vi "SRS cleanup.vi"(8 "error in (no error)":errorcluster, 11 "RUS settings":T1={"NI-DAQ lockin settings"={"Samples per sine wave"=0, "Sine waves per freq step"=0, "Output Representation"=enum."Real/Imaginary", "Low-pass filter"=enum."Butterworth", "Ranges and couplings "=[]}, "Fast swep settings"={"Update rate (Hz)"=250.0, "Start F, Hz"=200000.0, "Stop F"=1700000.0, "Number of points"=30000, "Amplitude"=2.1, "Init&amplitude"=TRUE, "IF"=1000.0, "Time constant"=0.1}, "Pre-sweep delay, s"=0.0, "Lockin mode"=enum."NI-DAQ", "SR Lockin"="GPIB0::10::INSTR", "DAQmx Device"="Dev3", "Clock Multiplier"=64, "Fast Sweep Data Out"={"DO clock task"="", "DO task"="", "Update clock task"="", "DAQ lockin task"="", "Pre-sweep counter task"=""}, "Lockin Range, V"=0.0, "F Array"=[], "Freq. update clock terminal"="", "DO Clock Rate (Hz)"=5000000.0, "ADC clock terminal"="/PFI4", "Pre-sweep counter terminal"="/PFI4", "Samples per read"=10, "DO clock terminal"="", "Pre-sweep points"=0, "F points per write"=0, "Total sweep time, s"=1000.0, "Initial SYNTH phase"=0.0, "Record IF"=FALSE, "Save data settings"={"Save data"=TRUE, "Data Root Path"=path "", "File Prefix"="", "File Format"=enum."ASCII", "Save column names"=TRUE, "File Comments"="<Description of the current file>", "User/Prj"="<User Name/Project Description>"}, "Data file path"=path "", "New data user event"=refnum, "Stop user event"=refnum, "Number of channels"=1, "Auto-phase"=FALSE} {"Lockin Range, V" format="%#_6e"; "Fast swep settings"."IF" format="%#_6p"; "Fast swep settings"."Amplitude" min=0.0 max=2.5; "Fast swep settings"."Number of points" format="%.0p"; "Fast swep settings"."Stop F" format="%#_6p"; "Fast swep settings"."Start F, Hz" format="%#_6p"; "Fast swep settings"."Update rate (Hz)" format="%0.2f"; "NI-DAQ lockin settings"."Ranges and couplings"."Coupling" items=["default"=-1, "RSE"=10083, "NRSE"=10078, "Differential"=10106, "Pseudodifferential"=12529]}) -> (0 "error out":errorcluster, 3 "VISA resource name out":refnum<visa-resource-name>, 4 "STD status byte":u8 format="%08b", 5 "Error status byte\n(bit 5 - FAST aborted)":u8 format="%08b")   [LabVIEW 2015]
uses:
  resonant_ultrasound/Libraries/RUS/Controls/RUS settings.ctl
  resonant_ultrasound/Libraries/RUS/Controls/RUS NI-DAQ Lockin Settings.ctl
  resonant_ultrasound/Libraries/RUS/Controls/Sweep settings.ctl
  File/Controls/Save data settings.ctl
  File/Controls/File formats.ctl
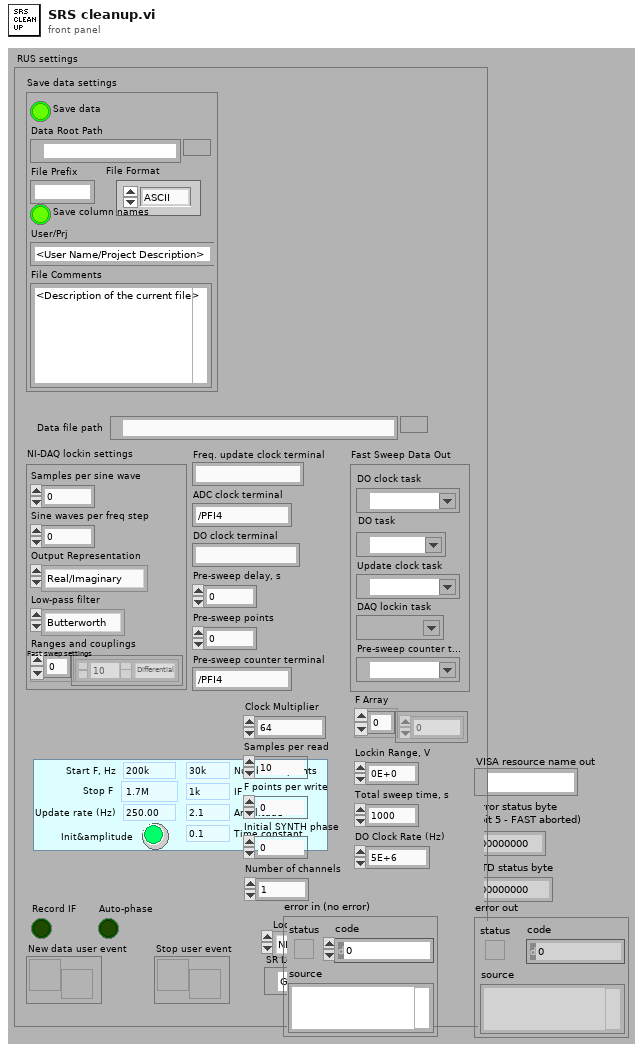
[diagram p1: front panel]
types:
  T1 = typedef "RUS settings.ctl" = cluster{"NI-DAQ lockin settings":T2, "Fast swep settings":T3, "Pre-sweep delay, s":dbl, "Lockin mode":enum16{"SRS", "NI-DAQ"}, "SR Lockin":refnum<visa-resource-name>, "DAQmx Device":tag, "Clock Multiplier":i32, "Fast Sweep Data Out":cluster{"DO clock task":refnum<k21>, "DO task":refnum<k21>, "Update clock task":refnum<k21>, "DAQ lockin task":refnum<k21>, "Pre-sweep counter task":refnum<k21>}, "Lockin Range, V":sgl, "F Array":dbl[], "Freq. update clock terminal":string, "DO Clock Rate (Hz)":dbl, "ADC clock terminal":string, "Pre-sweep counter terminal":string, "Samples per read":i32, "DO clock terminal":string, "Pre-sweep points":i32, "F points per write":i32, "Total sweep time, s":dbl, "Initial SYNTH phase":dbl, "Record IF":bool, "Save data settings":T4, "Data file path":path, "New data user event":refnum<user-event>, "Stop user event":refnum<user-event>, "Number of channels":i32, "Auto-phase":bool}
  T2 = typedef "RUS NI-DAQ Lockin Settings.ctl" = cluster{"Samples per sine wave":i32, "Sine waves per freq step":i32, "Output Representation":enum16{"Real/Imaginary", "Polar"}, "Low-pass filter":enum16{"No filtering", "Butterworth", "Bessel"}, "Ranges and couplings ":cluster{"Range":dbl, "Coupling":i32}[]}
  T3 = typedef "Sweep settings.ctl" = cluster{"Update rate (Hz)":dbl, "Start F, Hz":dbl, "Stop F":dbl, "Number of points":i32, "Amplitude":dbl, "Init&amplitude":bool, "IF":dbl, "Time constant":dbl}
  T4 = typedef "Save data settings.ctl" = cluster{"Save data":bool, "Data Root Path":path, "File Prefix":string, "File Format":T5, "Save column names":bool, "File Comments":string, "User/Prj":string}
  T5 = typedef "File formats.ctl" = enum16{"TDMS", "ASCII", "BINARY"}
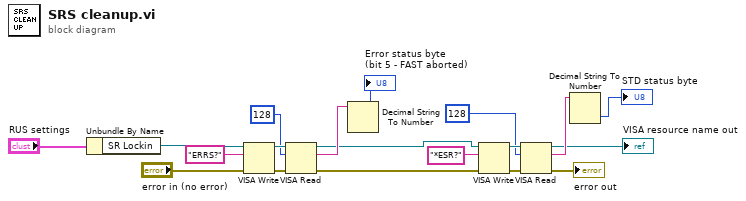
[diagram p0: block diagram]
diagram:
  n1 = Unbundle By Name("RUS settings") -> ("SR Lockin"=w1:refnum<visa-resource-name>)
  n2 = VISA Write(VISA resource name=w1, write buffer="ERRS?", error in (no error)="error in (no error)") -> (VISA resource name out=w17:refnum<visa-resource-name>, error out=w19:errorcluster)  [unwired: 1 out]
  n3 = VISA Read(VISA resource name=w17, byte count=u32 128, error in (no error)=w19) -> (VISA resource name out=w9:refnum<visa-resource-name>, read buffer=w14:string, error out=w8:errorcluster)  [unwired: 1 out]
  n4 = Decimal String To Number(string=w14) -> (number=→"Error status byte\n(bit 5 - FAST aborted)":i32)  [unwired: 3 out]
  n5 = VISA Write(VISA resource name=w9, write buffer="*ESR?", error in (no error)=w8) -> (VISA resource name out=w11:refnum<visa-resource-name>, error out=w13:errorcluster)  [unwired: 1 out]
  n6 = VISA Read(VISA resource name=w11, byte count=u32 128, error in (no error)=w13) -> (VISA resource name out=→"VISA resource name out":refnum<visa-resource-name>, read buffer=w10:string, error out=→"error out":errorcluster)  [unwired: 1 out]
  n7 = Decimal String To Number(string=w10) -> (number=→"STD status byte":i32)  [unwired: 3 out]
